vi "lab6-dev.vi"() -> ()   [LabVIEW 2015]
panel:
  in  "Valve Rate":i32(knob) scale=0.0..100.0
  out "Level Reached Alarm":bool
  in  "Desired Fill Level":dbl
  in  "Select Tank":dbl
  in  "On/Off":bool
  out "Tank 3":i32(slide) scale=0.0..1000.0
  out "Tank 2":i32(slide) scale=0.0..1000.0
  out "Tank":i32(slide) scale=0.0..1000.0
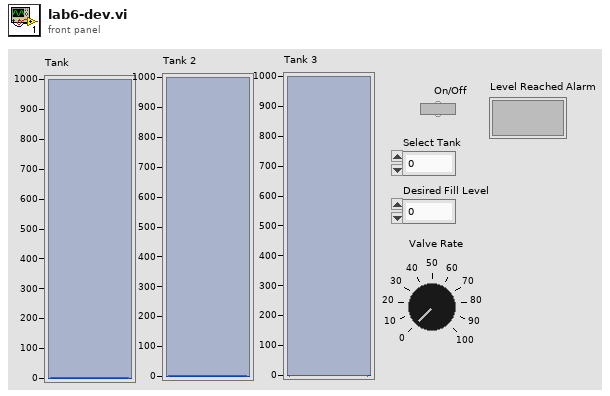
[diagram p1: front panel]
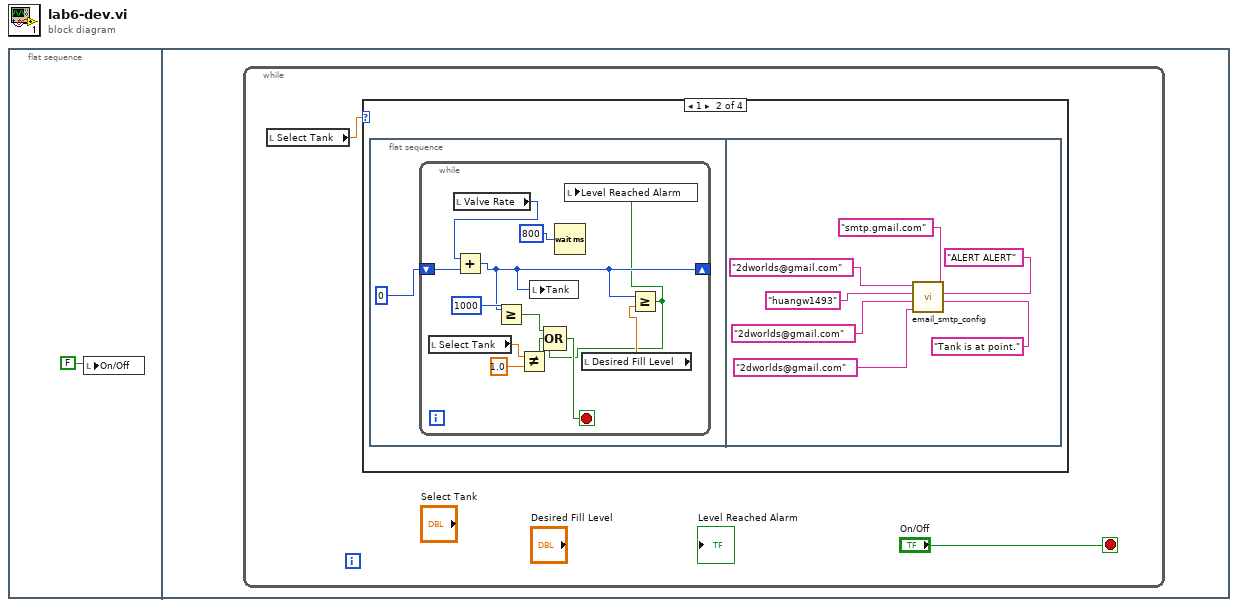
[diagram p0: block diagram]
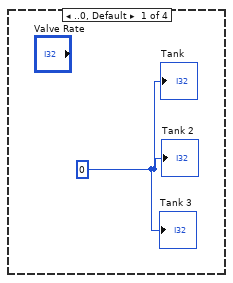
[diagram p2: hidden frame]
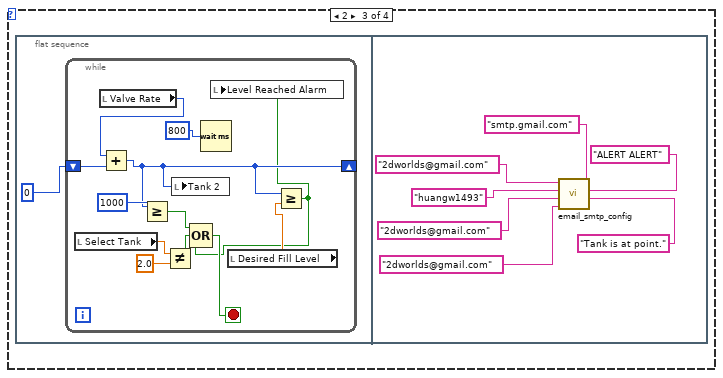
[diagram p3: hidden frame]
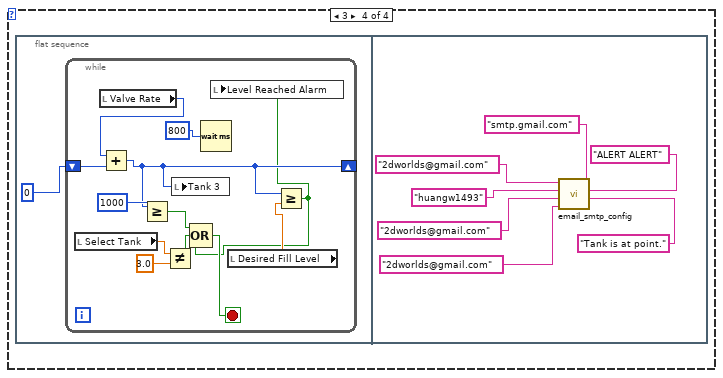
[diagram p4: hidden frame]
diagram:
  n1 = flat-sequence {
    frame #0 {
      n2 = local write "On/Off"(FALSE) -> ()
    }
    frame #1 {
      n3 = while {
        stop <- "On/Off" stop-if-true
        n4 = local read "Select Tank"() -> (w2:dbl)
        n5 = case shown="1" w2 {
          frame ..0, Default {
            w4 = 0
            "Tank 3" <- w4
            "Tank" <- w4
            "Tank 2" <- w4
          }
          frame 1 {
            n6 = flat-sequence {
              frame #0 {
                n7 = while {
                  shift-right: [w8] -> _
                  shift-left: 0 -> [w16]
                  stop <- w9 stop-if-true
                  n8 = local read "Select Tank"() -> (w13:dbl)
                  n9 = local read "Valve Rate"() -> (w14:i32)
                  n10 = Add(x=w14, y=w16) -> (x+y=w8:i32)
                  n11 = Greater Or Equal?(x=w8, y=1000) -> (x >= y?=w10:bool)
                  n12 = Not Equal?(x=w13, y=1.0) -> (x != y?=w11:bool)
                  n13 = local write "Tank"(w8) -> ()
                  n14 = Wait (ms)(milliseconds to wait=800) -> ()  [unwired: 1 out]
                  n15 = local read "Desired Fill Level"() -> (w7:dbl)
                  n16 = Greater Or Equal?(x=w8, y=w7) -> (x >= y?=w6:bool)
                  n17 = Compound Arithmetic op=OR(w10, w11, w6) -> (w9:bool)
                  n18 = local write "Level Reached Alarm"(w6) -> ()
                }
              }
              frame #1 {
                n19 = call "email_smtp_config.vi"("Body"="Tank is at point.", "Subject"="ALERT ALERT", "Outgoing Mail Server (SMTP)"="smtp.gmail.com", "Recipient's Email Address"="2dworlds@gmail.com", "Sender's Email Address"="2dworlds@gmail.com" ("GMAIL Account Password"), "GMAIL Account Password"="huangw1493", "GMAIL Account User ID"="2dworlds@gmail.com") -> ()  [unwired: 5 in]
              }
            }
          }
          frame 2 {
            n20 = flat-sequence {
              frame #0 {
                n21 = while {
                  shift-right: [w28] -> _
                  shift-left: 0 -> [w36]
                  stop <- w29 stop-if-true
                  n22 = local read "Select Tank"() -> (w33:dbl)
                  n23 = local read "Valve Rate"() -> (w34:i32)
                  n24 = Add(x=w34, y=w36) -> (x+y=w28:i32)
                  n25 = Greater Or Equal?(x=w28, y=1000) -> (x >= y?=w30:bool)
                  n26 = Not Equal?(x=w33, y=2.0) -> (x != y?=w31:bool)
                  n27 = local write "Tank 2"(w28) -> ()
                  n28 = Wait (ms)(milliseconds to wait=800) -> ()  [unwired: 1 out]
                  n29 = local read "Desired Fill Level"() -> (w27:dbl)
                  n30 = Greater Or Equal?(x=w28, y=w27) -> (x >= y?=w26:bool)
                  n31 = Compound Arithmetic op=OR(w30, w31, w26) -> (w29:bool)
                  n32 = local write "Level Reached Alarm"(w26) -> ()
                }
              }
              frame #1 {
                n33 = call "email_smtp_config.vi"("Body"="Tank is at point.", "Subject"="ALERT ALERT", "Outgoing Mail Server (SMTP)"="smtp.gmail.com", "Recipient's Email Address"="2dworlds@gmail.com", "Sender's Email Address"="2dworlds@gmail.com" ("GMAIL Account Password"), "GMAIL Account Password"="huangw1493", "GMAIL Account User ID"="2dworlds@gmail.com") -> ()  [unwired: 5 in]
              }
            }
          }
          frame 3 {
            n34 = flat-sequence {
              frame #0 {
                n35 = while {
                  shift-right: [w48] -> _
                  shift-left: 0 -> [w56]
                  stop <- w49 stop-if-true
                  n36 = local read "Select Tank"() -> (w53:dbl)
                  n37 = local read "Valve Rate"() -> (w54:i32)
                  n38 = Add(x=w54, y=w56) -> (x+y=w48:i32)
                  n39 = Greater Or Equal?(x=w48, y=1000) -> (x >= y?=w50:bool)
                  n40 = Not Equal?(x=w53, y=3.0) -> (x != y?=w51:bool)
                  n41 = local write "Tank 3"(w48) -> ()
                  n42 = Wait (ms)(milliseconds to wait=800) -> ()  [unwired: 1 out]
                  n43 = local read "Desired Fill Level"() -> (w47:dbl)
                  n44 = Greater Or Equal?(x=w48, y=w47) -> (x >= y?=w46:bool)
                  n45 = Compound Arithmetic op=OR(w50, w51, w46) -> (w49:bool)
                  n46 = local write "Level Reached Alarm"(w46) -> ()
                }
              }
              frame #1 {
                n47 = call "email_smtp_config.vi"("Body"="Tank is at point.", "Subject"="ALERT ALERT", "Outgoing Mail Server (SMTP)"="smtp.gmail.com", "Recipient's Email Address"="2dworlds@gmail.com", "Sender's Email Address"="2dworlds@gmail.com" ("GMAIL Account Password"), "GMAIL Account Password"="huangw1493", "GMAIL Account User ID"="2dworlds@gmail.com") -> ()  [unwired: 5 in]
              }
            }
          }
        }
      }
    }
  }
